vi "ReadCamCalibFile.vi"(8 "error in (no error)":errorcluster, 11 "Spec_Calib_file in":path) -> (0 "error out":errorcluster, 3 "Cam Calib Array":T1[](array[typedef]))   [LabVIEW 2020]
uses:
  CameraSettings_File.ctl
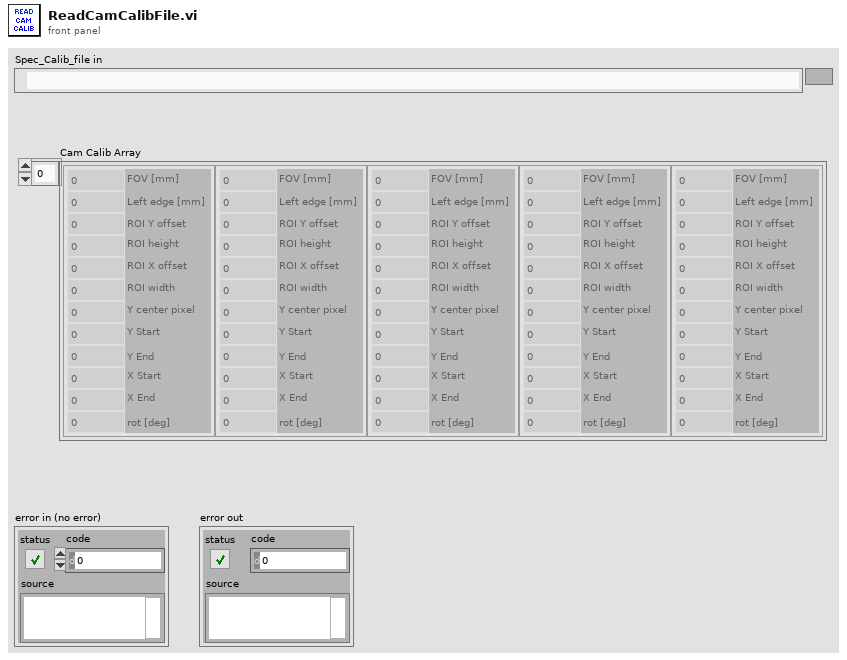
[diagram p1: front panel]
types:
  T1 = typedef "CameraSettings_File.ctl" = cluster{"FOV [mm]":dbl, "Left edge [mm]":dbl, "ROI Y offset":dbl, "ROI height":dbl, "ROI X offset":dbl, "ROI width":dbl, "Y center pixel":dbl, "Y Start":dbl, "Y End":dbl, "X Start":dbl, "X End":dbl, "rot [deg]":dbl}
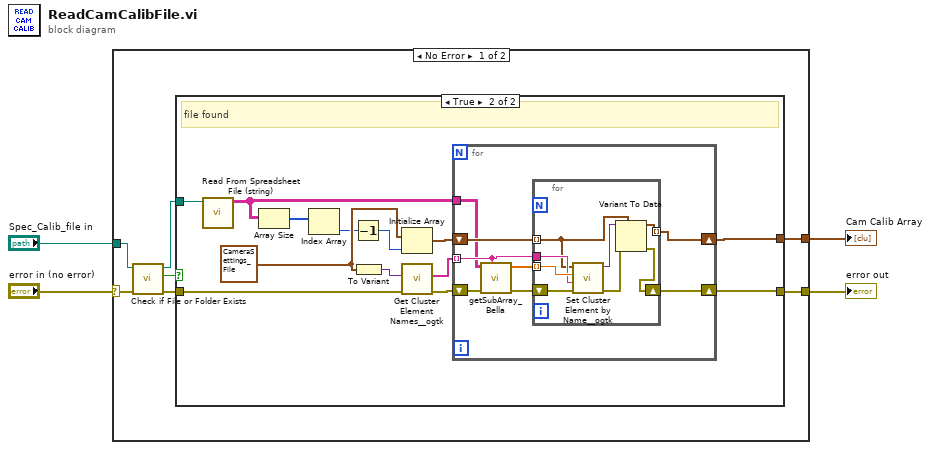
[diagram p0: block diagram]
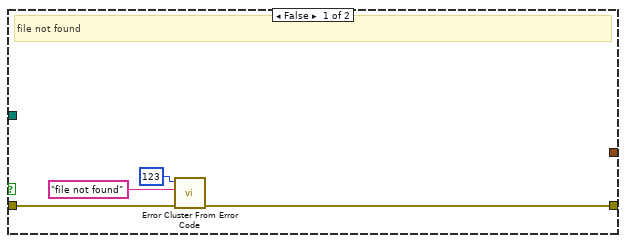
[diagram p2: hidden frame]
diagram:
  n1 = case shown="No Error" "error in (no error)" {
    selector: "error in (no error)" -> [w6 w45]
    tunnel: [w11 w45] -> w4
    tunnel: [w10 _] -> w1
    tunnel: "Spec_Calib_file in" -> [w7 _]
    frame No Error {
      n2 = call "Check if File or Folder Exists.vi"("error in (no error)"=w6, "path"=w7) -> ("error out"=w9:errorcluster, "file or folder exists?"=w5:bool, "dup path"=w8:path)  [unwired: 7 in]
      n3 = case shown="True" w5 {
        tunnel: [w12 w16] -> w11
        tunnel: [_ w17] -> w10
        tunnel: w9 -> [w13 w25]
        tunnel: w8 -> [_ w24]
        frame False {
          # "file not found"
          n4 = call "Error Cluster From Error Code.vi"("error in (no error)"=w13, "error message (\"\")"="file not found" ("source"), "error code (0)"=123 ("code")) -> ("error out"=w12:errorcluster)  [unwired: 6 in]
        }
        frame True {
          w23 = T1 {"FOV [mm]"=0.0, "Left edge [mm]"=0.0, "ROI Y offset"=0.0, "ROI height"=0.0, "ROI X offset"=0.0, "ROI width"=0.0, "Y center pixel"=0.0, "Y Start"=0.0, "Y End"=0.0, "X Start"=0.0, "X End"=0.0, "rot [deg]"=0.0}
          # "file found"
          n5 = call "Read From Spreadsheet File (string).vi"("file path (dialog if empty)"=w24) -> ("all rows"=w22:string[][])  [unwired: 6 in, 4 out]
          n6 = Array Size(array=w22) -> (size(s)=w21:i32[])
          n7 = Index Array(array=w21) -> (element=w20:i32)  [unwired: 1 in]
          n8 = Decrement(x=w20) -> (x-1=w19:i32)
          n9 = To Variant(anything=w23) -> (Variant=w26:variant)
          n10 = Initialize Array(w23, w19) -> (w18:T1[])
          n11 = call "Get Cluster Element Names__ogtk.vi"("error in (no error)"=w25, "Cluster"=w26) -> ("error out"=w28:errorcluster, "Element Names"=w27:string[])  [unwired: 8 in]
          n12 = for {
            tunnel: w22 -> [w31]
            tunnel: w27 -> [w33] mode=indexing
            shift-right: [w35] -> w16
            shift-left: w28 -> [w30]
            shift-right: [w34] -> w17
            shift-left: w18 -> [w36]
            n13 = call "getSubArray_Bella.vi"("element"=w33, "error in (no error)"=w30, "Array IN"=w31) -> ("error out"=w29:errorcluster, "Array out"=w32:dbl[])  [unwired: 7 in]
            n14 = for {
              tunnel: w32 -> [w44] mode=indexing
              tunnel: w33 -> [w42]
              tunnel: w36 -> [w40] mode=indexing
              shift-right: [w37] -> w35
              shift-left: w29 -> [w43]
              tunnel: [w39] -> w34 mode=indexing
              n15 = call "Set Cluster Element by Name__ogtk.vi"("error in (no error)"=w43, "Element Name (\"\": New Element Data Name)"=w42, "New Element Value"=w44, "Cluster"=w40) -> ("error out"=w38:errorcluster, "VCluster out"=w41:variant)  [unwired: 5 in, 1 out]
              n16 = Variant To Data(error in=w38, type=w40, Variant=w41) -> (data=w39:T1, error out=w37:errorcluster)
            }
          }
        }
      }
    }
    frame Error {
    }
  }
  "error out" <- w4
  "Cam Calib Array" <- w1
